vi "oa_TV Update Angle interval (NChan).vi"(5 "reset? (F)":bool, 8 "error in (no error)":errorcluster, 9 "pulse/revolution":i32[](array[numeric]), 10 "revulotion index":i32[](array[numeric]), 11 "pulse position [s]":cluster{dbl[]}[](array[cluster]) {"?" format="%.2f"}) -> (0 "error out":errorcluster, 3 "angle intervals":cluster{dbl[]}[](array[cluster]))   [LabVIEW 2017, in "SoundVib_Torsional.lvlib"]
uses:
  <vilib>/addons/Sound and Vibration/Order Analysis/Torsional Vibration/SoundVib_Torsional.lvlib
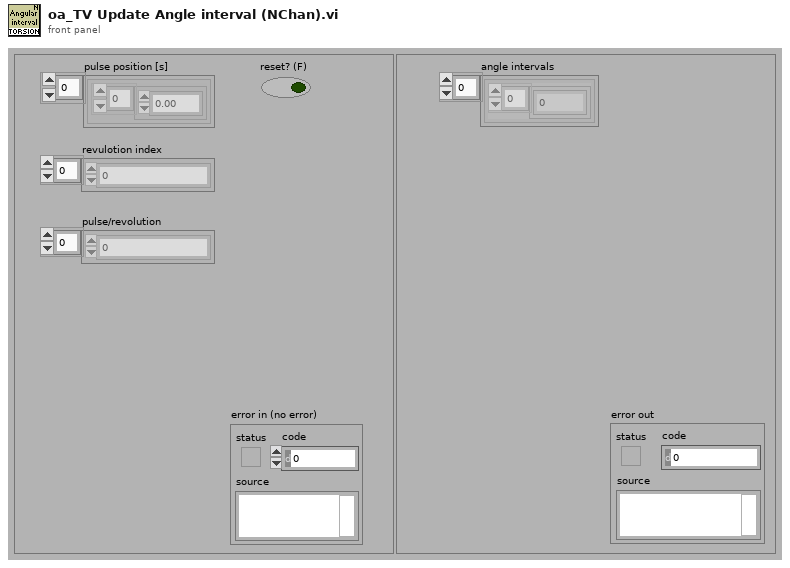
[diagram p1: front panel]
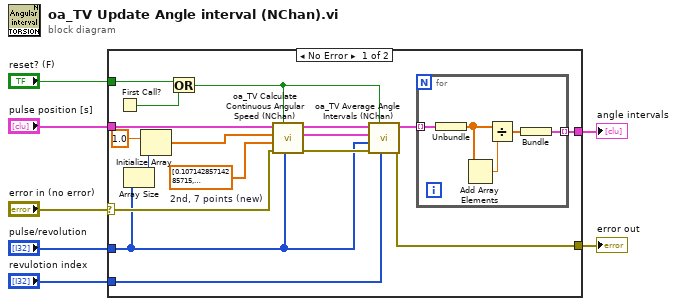
[diagram p0: block diagram]
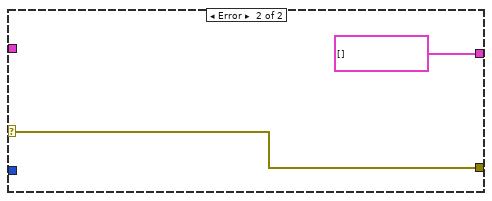
[diagram p2: hidden frame]
diagram:
  n1 = case shown="No Error" "error in (no error)" {
    selector: "error in (no error)" -> [w19 w31]
    tunnel: "revulotion index" -> [w13 _]
    tunnel: [w23 cluster{dbl[]}[] []] -> w2
    tunnel: [w22 w31] -> w6
    tunnel: "pulse/revolution" -> [w12 _]
    tunnel: "pulse position [s]" -> [w17 _]
    tunnel: "reset? (F)" -> [w8 _]
    frame No Error {
      w20 = dbl[] [0.10714285714285715, 0.07142857142857142, 0.035714285714285705, -1.5209319782164736e-17, -0.03571428571428571, -0.07142857142857142, -0.10714285714285715]  # 2nd, 7 points (new)
      n2 = First Call?() -> (First Call?: T/F=w24:bool)
      n3 = Array Size(array=w12) -> (size(s)=w15:i32)
      n4 = Initialize Array(1.0 ("deltaX"), w15) -> (w14:dbl[])
      n5 = Or(x=w8, y=w24) -> (x .or. y?=w21:bool)
      n6 = call <vilib>:"oa_TV Calculate Continuous Angular Speed (NChan).vi"("pulse/revolution (1)"=w12, "reset? (False)"=w21, "error in (no error)"=w19, "filter coefficients"=w20, "deltaX"=w14, "Y[n]"=w17) -> ("error out"=w18:errorcluster, "dY[n]/dX[n]"=w10:cluster{dbl[]}[], "pulse out"=w11:cluster{dbl[]}[])  [unwired: 3 in]
      n7 = call <vilib>:"oa_TV Average Angle Intervals (NChan).vi"("revulotion index"=w13, "reset? (F)"=w21, "error in (no error)"=w18, "pulse/revolution"=w12, "RPM"=w10, "time index"=w11) -> ("error out"=w22:errorcluster, "angle intervals"=w9:cluster{"angle intervals":dbl[]}[])  [unwired: 4 in]
      n8 = for {
        tunnel: [w25] -> w23 mode=indexing
        tunnel: w9 -> [w28] mode=indexing
        n9 = Unbundle(w28) -> ("angle intervals"=w27:dbl[])
        n10 = Add Array Elements(numeric array=w27) -> (sum=w29:dbl)
        n11 = Divide(x=w27, y=w29) -> (x/y=w26:dbl[])
        n12 = Bundle(w26) -> (w25:cluster{dbl[]})  [unwired: 1 in]
      }
    }
    frame Error {
    }
  }
  "error out" <- w6
  "angle intervals" <- w2
